vi "Test Find Chessboard Corners Sector Based.vi"(8 "error in (no error)":errorcluster, 11 "Test Case In":refnum<class "CameraCalibration.lvclass">) -> (0 "error out":errorcluster, 3 "Test Case Out":refnum<class "CameraCalibration.lvclass">)   [LabVIEW 2020, in "test.lvlib" / "CameraCalibration.lvclass"]
uses:
  CameraCalibration.lvclass
  C:/Program Files (x86)/National Instruments/LabVIEW 2020/vi.lib/Astemes/LUnit/Test Case.lvclass
  feature_detection/Find Chessboard Corners Sector Based Flags.ctl
  common/Image Size (Integer).ctl
  feature_detection/Chessboard Corner Info.ctl
  common/Image Point (Float).ctl
  <vilib>/Astemes/LUnit/Test Case.lvclass/Test Case.ctl
  image/Line Type.ctl
  image/New Image (Greyscale).vi
  image/Copy Pixmap to Image (Greyscale Flatten Mask).vi
  feature_detection/FindChessboardCornersSectorBasedGreyscale.vi
  image/Draw Circle (Greyscale).vi
  image/Draw Rectangle (Greyscale).vi
  image/Draw Image to Picture (Greyscale).vi
  feature_detection/DrawChessboardSemiCircleSquare.vi
  feature_detection/DrawChessboardTearDropSquare.vi
  feature_detection/DrawChessboardSpotOnSquare.vi
  feature_detection/DrawChessboardRadon.vi/e7f4303d-582b-4721-b29a-aa63d9231187.vi
  image/New Image (Greyscale).vi/6598b9e0-8a08-46f5-91fd-ca1b87217137.vi
  image/Copy Pixmap to Image (Greyscale Flatten Mask).vi/f0818824-bd55-4656-87f2-fcc208e7cf24.vi
  feature_detection/FindChessboardCornersSectorBasedGreyscale.vi/6a9761e7-0504-45a6-89a0-1e961674e9fc.vi
  <vilib>/Astemes/LUnit/Append Fail Result.vi
  <vilib>/Astemes/LUnit/Append Pass Result.vi
  image/Draw Circle (Greyscale).vi/8336a1cf-e433-4bea-8080-376bdb783d4e.vi
  image/Draw Rectangle (Greyscale).vi/7e6fb015-3761-4366-a0a7-e436eb229083.vi
  image/Draw Image to Picture (Greyscale).vi/9ae995ca-ccda-485c-89ac-02736fde3e8e.vi
  image/FixPixmap.vi
  <vilib>/Astemes/LUnit/Run In UI.vi
  image/Default8bitColourMap.vi
  <vilib>/Utility/error.llb/Clear Errors.vi
  <vilib>/picture/picture.llb/Draw Oval.vi
  <vilib>/picture/picture.llb/Draw Rectangle.vi
  <vilib>/picture/pictutil.llb/Picture to Pixmap.vi
  common/Module Path.vi
  <vilib>/Utility/error.llb/Error Cluster From Error Code.vi
  <vilib>/Comparison/Equal/Equal Functor/Equal Functor.lvclass
  image/image.lvlib
  feature_detection/feature_detection.lvlib
  <vilib>/Astemes/LUnit/Test Case.lvclass
  common/common.lvlib
panel:
  out "Picture":picture
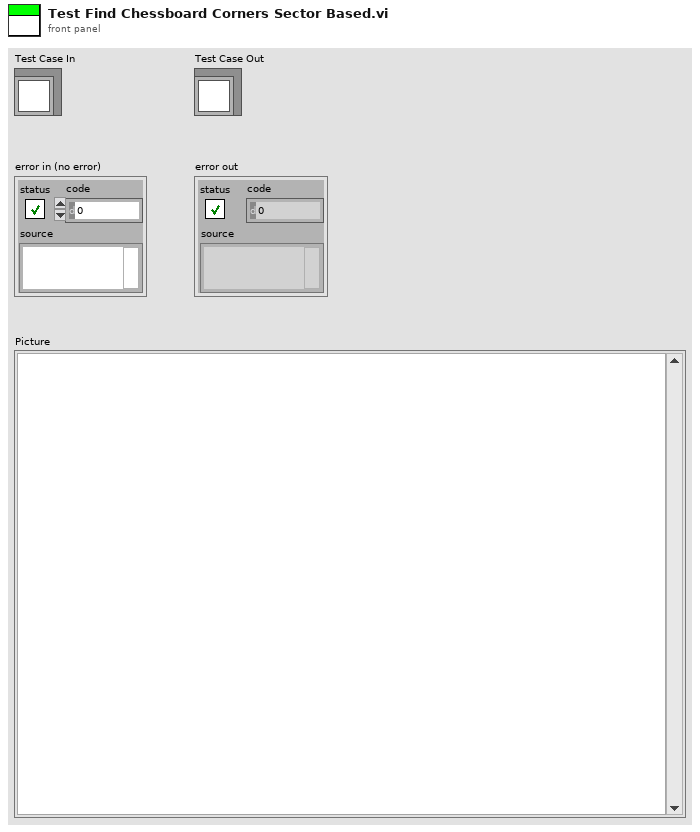
[diagram p1: front panel]
types:
  T1 = typedef "common.lvlib/Image Point (Float).ctl" = cluster{"x":dbl, "y":dbl}
  T2 = typedef "feature_detection.lvlib/Chessboard Corner Info.ctl" = cluster{"Points Per Row":u8, "Points Per Col":u8}
  T3 = typedef "common.lvlib/Image Size (Integer).ctl" = cluster{"Width":u16, "Height":u16}
  T4 = typedef "feature_detection.lvlib/Find Chessboard Corners Sector Based Flags.ctl" = enum16{"CALIB_CB_NORMALIZE_IMAGE", "CALIB_CB_EXHAUSTIVE", "CALIB_CB_ACCURACY", "CALIB_CB_LARGER", "CALIB_CB_MARKER"}
  T5 = typedef "imagedata.ctl" = cluster{"image type":i32, "image depth":i32, "image":u8[], "mask":u8[], "colors":u32[], "Rectangle":cluster{"left":i16, "top":i16, "right":i16, "bottom":i16}}
  T6 = typedef "image.lvlib/Greyscale Image.ctl" = refnum<data-value>
  T7 = typedef "feature_detection.lvlib/Find Chessboard Corners Sector Based Meta.ctl" = enum16{"No Meta Data", "Left-Top Corner Black Cell", "Left-Top Corner White Cell", "Left-Top Corner Black Cell with Marker", "Left-Top Corner White Cell with Marker"}
  T8 = typedef "image.lvlib/Line Type.ctl" = enum8{"FILLED", "LINE_4", "LINE_8", "LINE_AA"}
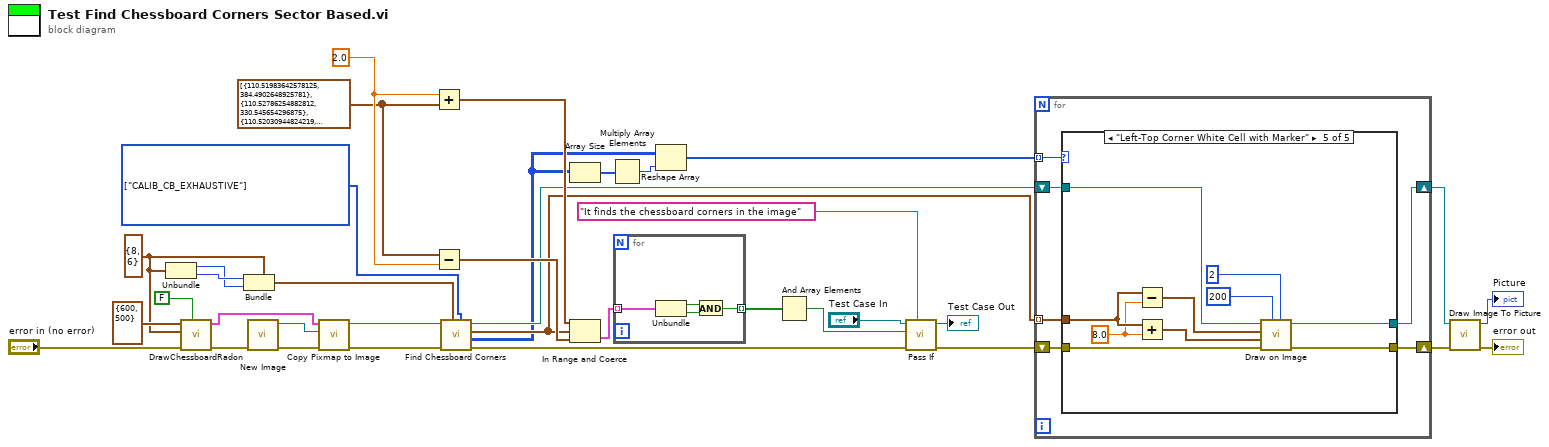
[diagram p0: block diagram]
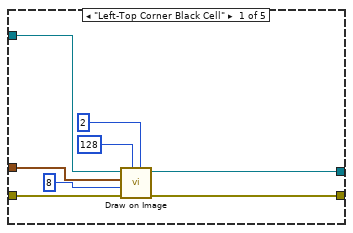
[diagram p2: hidden frame]
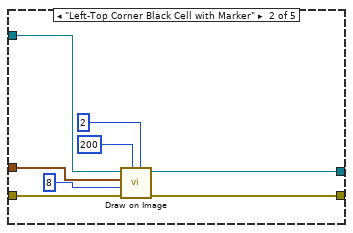
[diagram p3: hidden frame]
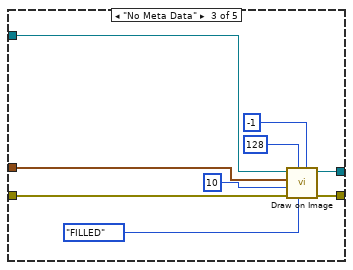
[diagram p4: hidden frame]
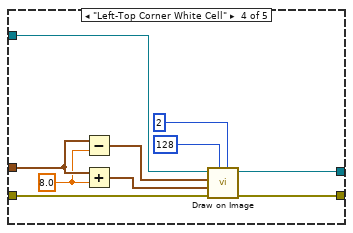
[diagram p5: hidden frame]
diagram:
  w3 = T1[] [{"x"=110.51983642578125, "y"=384.4902648925781}, {"x"=110.52786254882812, "y"=330.545654296875}, {"x"=110.52030944824219, "y"=276.5110168457031}, {"x"=110.52304077148438, "y"=222.49684143066406}, {"x"=110.52587127685547, "y"=168.5770263671875}, {"x"=110.5278549194336, "y"=114.48518371582031}, {"x"=164.4899139404297, "y"=384.4825744628906}, {"x"=164.49302673339844, "y"=330.5461730957031}, {"x"=164.4706268310547, "y"=276.5264892578125}, {"x"=164.47882080078125, "y"=222.49041748046875}, {"x"=164.487060546875, "y"=168.57138061523438}, {"x"=164.49017333984375, "y"=114.49085235595703}, {"x"=218.58425903320312, "y"=384.4807434082031}, {"x"=218.58438110351562, "y"=330.5576477050781}, {"x"=218.56167602539062, "y"=276.5283508300781}, {"x"=218.5755615234375, "y"=222.49874877929688}, {"x"=218.56430053710938, "y"=168.5651092529297}, {"x"=218.57057189941406, "y"=114.4876708984375}, {"x"=272.4980773925781, "y"=384.4714050292969}, {"x"=272.4951477050781, "y"=330.5459289550781}, {"x"=272.4820861816406, "y"=276.52618408203125}, {"x"=272.4815368652344, "y"=222.4823455810547}, {"x"=272.4978942871094, "y"=168.5762939453125}, {"x"=272.4895324707031, "y"=114.4795150756836}, {"x"=326.50860595703125, "y"=384.4912109375}, {"x"=326.507568359375, "y"=330.5517578125}, {"x"=326.52020263671875, "y"=276.52099609375}, {"x"=326.5254211425781, "y"=222.48287963867188}, {"x"=326.52752685546875, "y"=168.56243896484375}, {"x"=326.525634765625, "y"=114.47119903564453}, {"x"=380.5481262207031, "y"=384.49346923828125}, {"x"=380.5423278808594, "y"=330.5431213378906}, {"x"=380.5509948730469, "y"=276.5083312988281}, {"x"=380.5451354980469, "y"=222.4959716796875}, {"x"=380.55682373046875, "y"=168.58506774902344}, {"x"=380.54541015625, "y"=114.49372100830078}, {"x"=434.4837646484375, "y"=384.4846496582031}, {"x"=434.4927062988281, "y"=330.54888916015625}, {"x"=434.49041748046875, "y"=276.5093688964844}, {"x"=434.4705810546875, "y"=222.49887084960938}, {"x"=434.4798889160156, "y"=168.5850067138672}, {"x"=434.4817810058594, "y"=114.49042510986328}, {"x"=488.5366516113281, "y"=384.4859619140625}, {"x"=488.5210876464844, "y"=330.5379638671875}, {"x"=488.5309143066406, "y"=276.51507568359375}, {"x"=488.5359191894531, "y"=222.48826599121094}, {"x"=488.5423278808594, "y"=168.5687713623047}, {"x"=488.54949951171875, "y"=114.49140167236328}] ("Points")
  w11 = T2 {"Points Per Row"=8, "Points Per Col"=6} ("Chessboard Corners Info")
  w2 = T4[] [enum."CALIB_CB_EXHAUSTIVE"] items=["CALIB_CB_NORMALIZE_IMAGE", "CALIB_CB_EXHAUSTIVE", "CALIB_CB_ACCURACY", "CALIB_CB_LARGER", "CALIB_CB_MARKER"] ("Flags (Default: None)")
  w36 = 2.0
  n1 = Unbundle(w11) -> ("Points Per Row"=w9:u8, "Points Per Col"=w10:u8)
  n2 = call "DrawChessboardRadon.vi"("Add Marker (Default: False)"=FALSE, "error in (no error)"="error in (no error)", "Chessboard Corners Info"=w11, "Target Size"=T3 {"Width"=600, "Height"=500}) -> ("error out"=w21:errorcluster, "image data"=w22:T5)  [unwired: 6 in]
  n3 = Bundle(cluster=w11, "Points Per Row"=w10, "Points Per Col"=w9) -> (w1:T2)
  n4 = call-poly "New Image.vi"("error in (no error)"=w21) -> ("error out"=w20:errorcluster, "New Greyscale Image"=w23:T6)  [unwired: 9 in]
  n5 = call-poly "Copy Pixmap to Image.vi"("error in (no error)"=w20, "Greyscale Image Destination"=w23, "Pixmap Image Data"=w22) -> ("error out"=w19:errorcluster, "Greyscale Image Destination (duplicate)"=w18:T6)  [unwired: 7 in]
  n6 = Add(x=w36, y=w3) -> (x+y=w31:T1[])
  n7 = Subtract(x=w3, y=w36) -> (x-y=w32:T1[])
  n8 = call-poly "Find Chessboard Corners.vi"("Flags (Default: None)"=w2, "Chessboard Corners Info"=w1, "error in (no error)"=w19, "Greyscale Image"=w18) -> ("error out"=w35:errorcluster, "Meta Data"=w7:T7[][], "Points"=w8:T1[], "Greyscale Image (Duplicate)"=w16:T6)  [unwired: 4 in]
  n9 = Array Size(array=w7) -> (size(s)=w6:i32[])
  n10 = In Range and Coerce(upper limit=w31, x=w8, lower limit=w32) -> (In Range?=w30:cluster{"x":bool, "y":bool}[])  [unwired: 1 out]
  n11 = Multiply Array Elements(1:w6) -> (0:w5:i32)
  n12 = for {
    tunnel: w30 -> [w40] mode=indexing
    tunnel: [w37] -> w29 mode=indexing
    n13 = Unbundle(w40) -> ("x"=w39:bool, "y"=w38:bool)
    n14 = And(x=w39, y=w38) -> (x .and. y?=w37:bool)
  }
  n15 = Reshape Array(w7, w5) -> (w4:T7[])
  n16 = And Array Elements(Boolean array=w29) -> (logical AND=w28:bool)
  n17 = call <vilib>:"Pass If.vi"("Description"="It finds the chessboard corners in the image", "error in (no error)"=w35, "Pass?"=w28, "LUnit Test Case In"="Test Case In") -> ("error out"=w14:errorcluster, "LUnit Test Case Out"=→"Test Case Out":refnum<class "CameraCalibration.lvclass">)  [unwired: 6 in]
  n18 = for {
    shift-right: [w43] -> w15
    shift-left: w16 -> [w46]
    shift-right: [w44] -> w13
    shift-left: w14 -> [w45]
    tunnel: w8 -> [w42] mode=indexing
    tunnel: w4 -> [w41] mode=indexing
    n19 = case shown="\"Left-Top Corner White Cell with Marker\"" w41 {
      tunnel: w46 -> [w54 w62 w71 w81 w91]
      tunnel: w45 -> [w53 w61 w70 w80 w90]
      tunnel: [w52 w60 w69 w79 w89] -> w44
      tunnel: [w51 w59 w68 w78 w88] -> w43
      tunnel: w42 -> [w50 w58 w67 w76 w86]
      frame "Left-Top Corner Black Cell" {
        n20 = call-poly "Draw on Image.vi"("Thickness (Default: 1)"=2, "Colour"=u8 128, "error in (no error)"=w53, "Radius"=u16 8, "Centre"=w50, "Greyscale Image"=w54) -> ("error out"=w52:errorcluster, "Greyscale Image (Duplicate)"=w51:T6)  [unwired: 4 in]
      }
      frame "Left-Top Corner Black Cell with Marker" {
        n21 = call-poly "Draw on Image.vi"("Thickness (Default: 1)"=2, "Colour"=u8 200, "error in (no error)"=w61, "Radius"=u16 8, "Centre"=w58, "Greyscale Image"=w62) -> ("error out"=w60:errorcluster, "Greyscale Image (Duplicate)"=w59:T6)  [unwired: 4 in]
      }
      frame "No Meta Data" {
        n22 = call-poly "Draw on Image.vi"("Thickness (Default: 1)"=-1, "OpenCV Line Type (Default LINE_8)"=Line_Type."FILLED", "Colour"=u8 128, "error in (no error)"=w70, "Radius"=u16 10, "Centre"=w67, "Greyscale Image"=w71) -> ("error out"=w69:errorcluster, "Greyscale Image (Duplicate)"=w68:T6)  [unwired: 3 in]
      }
      frame "Left-Top Corner White Cell" {
        w75 = 8.0
        n23 = Subtract(x=w76, y=w75) -> (x-y=w77:T1)
        n24 = Add(x=w76, y=w75) -> (x+y=w74:T1)
        n25 = call-poly "Draw on Image.vi"("Thickness (Default: 1)"=2, "Colour"=u8 128, "error in (no error)"=w80, "Point B"=w74, "Point A"=w77, "Greyscale Image"=w81) -> ("error out"=w79:errorcluster, "Greyscale Image (Duplicate)"=w78:T6)  [unwired: 4 in]
      }
      frame "Left-Top Corner White Cell with Marker" {
        w85 = 8.0
        n26 = Subtract(x=w86, y=w85) -> (x-y=w87:T1)
        n27 = Add(x=w86, y=w85) -> (x+y=w84:T1)
        n28 = call-poly "Draw on Image.vi"("Thickness (Default: 1)"=2, "Colour"=u8 200, "error in (no error)"=w90, "Point B"=w84, "Point A"=w87, "Greyscale Image"=w91) -> ("error out"=w89:errorcluster, "Greyscale Image (Duplicate)"=w88:T6)  [unwired: 4 in]
      }
    }
  }
  n29 = call-poly "Draw Image To Picture.vi"("error in (no error)"=w13, "Greyscale Image Source"=w15) -> ("error out"=→"error out":errorcluster, "Picture"=→"Picture":picture)  [unwired: 8 in]
